vi "TimeLine_Module.vi"(10 "문자열 입력":string) -> (2 "최근 타임라인":string, 3 "총 타임라인":string)   [LabVIEW 2020]
uses:
  <vilib>/Platform/TimedLoop/XDataNode/timing_clust.ctl
  <vilib>/Platform/TimedLoop/XDataNode/nitl_modes.ctl
  <vilib>/Platform/TimedLoop/XDataNode/wakeup.ctl
  var.vi
  <vilib>/Platform/TimedLoop/XDataNode/XDataNode.xnode
  <vilib>/Platform/TimedLoop/XDataNode/XDNodeRunTimeDep.lvlib
panel:
  in  "정지 버튼":bool
  # "2019243026 맹진영 작성"
  # "타임라인 기능 모듈의 테스트 케이스"
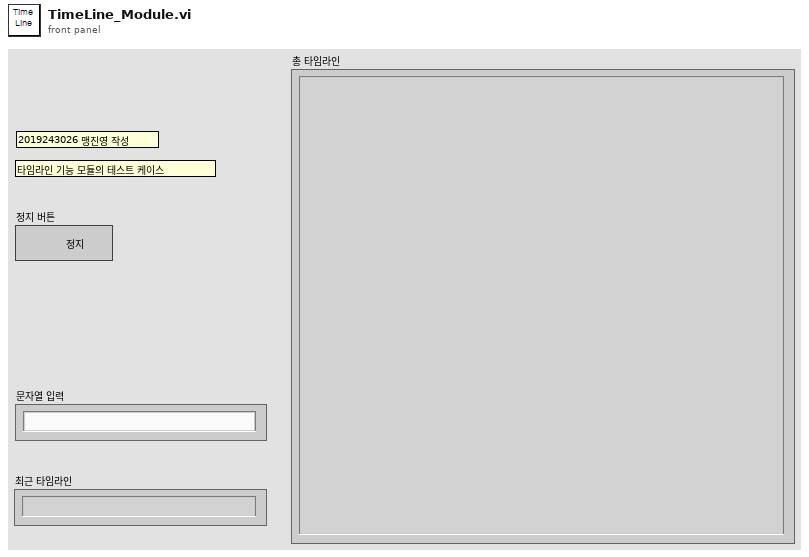
[diagram p1: front panel]
types:
  T1 = typedef "XDNodeRunTimeDep.lvlib/timing_clust.ctl" = cluster{"Expected End [f-1]":u64, "Actual End [f-1]":u64, "Finished Late? [f-1]":bool, "Expected End [i-1]":u64, "Actual End [i-1]":u64, "Finished Late? [i-1]":bool, "Expected Start [i]":u64, "Actual Start [i]":u64, "Expected Start [f]":u64, "Actual Start [f]":u64, "Source Name":string, "Structure Name":string, "Period":i64, "Deadline":i64, "Offset":i64, "Start":i64, "Priority":i32, "Timeout":i32, "Mode":T2, "Wakeup Reason":T3, "Error":errorcluster, "Source Type":string, "Secondary Source Type":string, "Global End Time":u64, "Global Start Time":u64, "Frame Duration":u64, "Iteration Duration":u64, "Assigned CPU":i32, "I/O Scan Engine Mode":u32}
  T2 = typedef "XDNodeRunTimeDep.lvlib/nitl_modes.ctl" = enum32{"No Change", "Process missed periods, maintain original phase", "Discard missed periods, maintain original phase", "Process missed periods, ignore original phase", "Discard missed periods, ignore original phase"}
  T3 = typedef "XDNodeRunTimeDep.lvlib/wakeup.ctl" = enum32{"Normal", "Aborted", "Asynchronous wakeup", "Timing source error", "Timed loop error", "Timeout"}
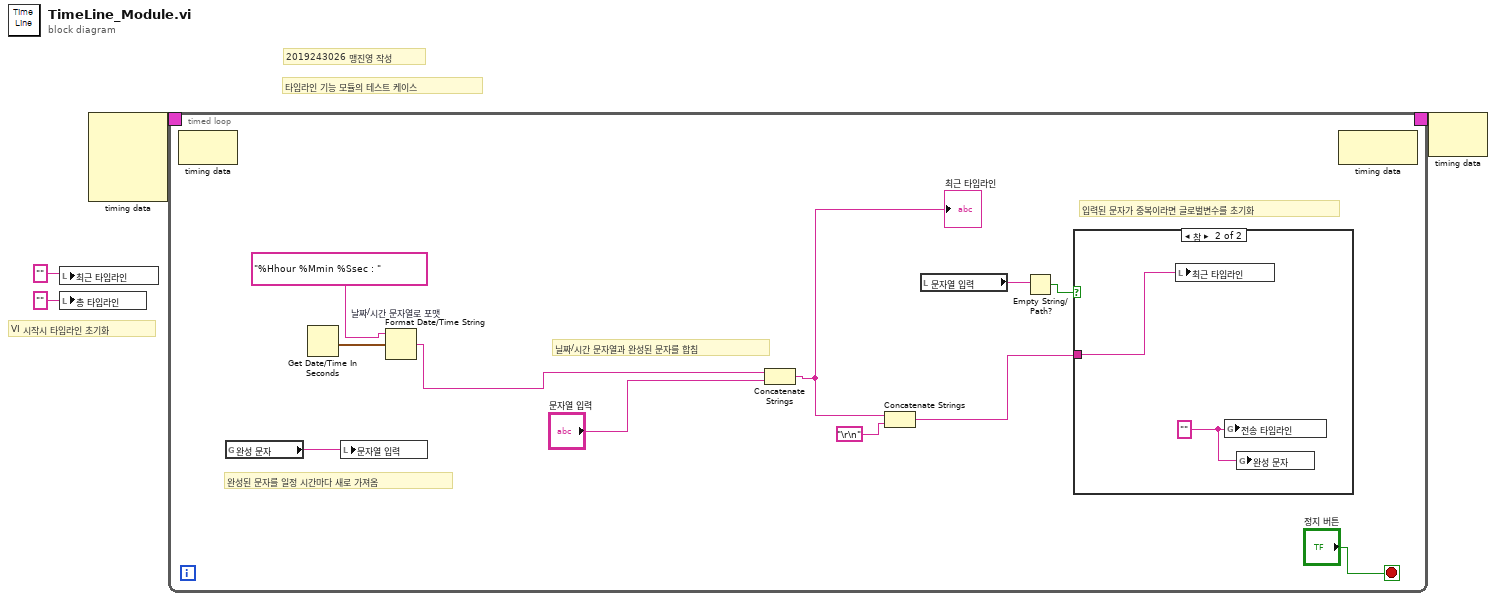
[diagram p0: block diagram]
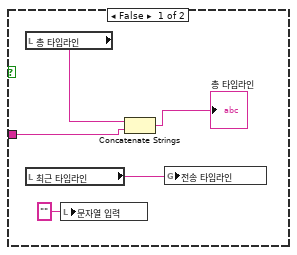
[diagram p2: hidden frame]
diagram:
  # "VI 시작시 타임라인 초기화"
  # "타임라인 기능 모듈의 테스트 케이스"
  # "2019243026 맹진영 작성"
  n1 = local write "최근 타임라인"("" ("최근 타임라인")) -> ()
  n2 = local write "총 타임라인"("") -> ()
  n3 = node-c288() -> (w2:T1)  [unwired: 4 in]
  n4 = timed-loop {
    timing: w2 -> [_]
    timing-out: [_] -> w1
    stop <- "정지 버튼" stop-if-true
    # "입력된 문자가 중복이라면 글로벌변수를 초기화"
    # "닐짜/시간 문자열과 완성된 문자를 합침"
    # "완성된 문자를 일정 시간마다 새로 가져옴"
    n5 = node-c288() -> ()  [unwired: 1 in, 1 out]
    n6 = global read "var.vi" "완성 문자"() -> (w11:string)
    n7 = Get Date/Time In Seconds() -> (seconds since 1Jan1904=w14:timestamp)
    n8 = local write "문자열 입력"(w11) -> ()
    n9 = Format Date/Time String "날짜/시간 문자열로 포맷"(time format string (%c)="%Hhour %Mmin %Ssec : ", seconds (now)=w14) -> (date/time string=w12:string)  [unwired: 1 in]
    n10 = Concatenate Strings(w12, "문자열 입력") -> (w6:string)
    "최근 타임라인" <- w6
    n11 = Concatenate Strings(w6, "\r\n") -> (w5:string)
    n12 = local read "문자열 입력"() -> (w8:string)
    n13 = Empty String/Path?(string/path=w8) -> (empty?=w7:bool)
    n14 = case shown="참" w7 {
      tunnel: w5 -> [w19 w22]
      frame False {
        n15 = local read "총 타임라인"() -> (w20:string)
        n16 = local read "최근 타임라인"() -> (w16:string)
        n17 = local write "문자열 입력"("" ("문자열 입력")) -> ()
        n18 = Concatenate Strings(w20, w19) -> (→"총 타임라인":string)
        n19 = global write "var.vi" "전송 타임라인"(w16) -> ()
      }
      frame True {
        w21 = "" ("문자열 입력")
        n20 = local write "최근 타임라인"(w22) -> ()
        n21 = global write "var.vi" "전송 타임라인"(w21) -> ()
        n22 = global write "var.vi" "완성 문자"(w21) -> ()
      }
    }
    n23 = node-c288() -> ()  [unwired: 1 in, 1 out]
  }
  n24 = node-c288(w1) -> ()  [unwired: 1 out]
